vi "Read JTAG Scan Chain IDCODEs.vi"() -> ()   [LabVIEW 2011, in "LVH-Adept.lvlib"]
uses:
  <vilib>/LabVIEW Hacker/Adept/LVH-Adept.lvlib
  <vilib>/LabVIEW Hacker/Adept/Private/Type Defs/Adept Device Ctl.xctl
panel:
  in  "Adept Device":u16(xcontrol)
  out "IDCODEs":u32[](array[numeric])
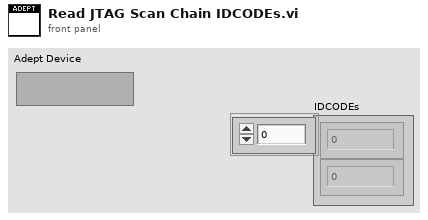
[diagram p1: front panel]
types:
  T1 = typedef "LVH-Adept.lvlib/Device Config.ctl" = cluster{"Num Devices":i32, "Device Names":string[], "Device Index":u16, "Device Handle":u32}
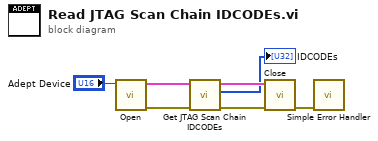
[diagram p0: block diagram]
diagram:
  n1 = call <vilib>:"Open.vi"("Adept Device Ctl"="Adept Device") -> ("Error Out"=w3:errorcluster, "Adept Config"=w7:T1)  [unwired: 9 in]
  n2 = call <vilib>:"Get JTAG Scan Chain IDCODEs.vi"("Error In"=w3, "Adept Device"=w7) -> ("Error In"=w5:errorcluster, "IDCODEs"=→"IDCODEs":u32[], "Adept Device"=w6:T1)  [unwired: 7 in]
  n3 = call <vilib>:"Close.vi"("Error In"=w5, "Adept Config"=w6) -> ("Error Out"=w1:errorcluster)  [unwired: 9 in]
  n4 = call <vilib>:"Simple Error Handler.vi"("error in (no error)"=w1) -> ()  [unwired: 4 in, 5 out]
